vi "Initialization.vi"(8 "error in (no error)":errorcluster, 9 "Init file":string="config_ligne_à_retard.ls", 11 "DelayLineLS4 in":refnum<class "DLLS4.lvclass">) -> (0 "error out":errorcluster, 3 "DelayLineLS4 out":refnum<class "DLLS4.lvclass">)   [LabVIEW 2018, in "DLLS4.lvclass"]
uses:
  DLLS4.lvclass
  C:/Users/Sergey Denisov/Documents/REPS/TRANCON/Classes/GeneralFunctionality/GeneralFunctionality.lvclass
  C:/Users/Sergey Denisov/Documents/REPS/TRANCON/Classes/Delay Line/DelayLine.lvclass
  GeneralFunctionality/GeneralFunctionality.lvclass/GeneralFunctionality.ctl
  DelayLine.lvclass/DelayLine.ctl
  dependecies/globalVarII.vi
  <vilib>/Utility/libraryn.llb/Check if File or Folder Exists.vi
  <vilib>/Utility/error.llb/Error Cluster From Error Code.vi
  Config/Config.lvclass
  DelayLine.lvclass
  GeneralFunctionality/GeneralFunctionality.lvclass
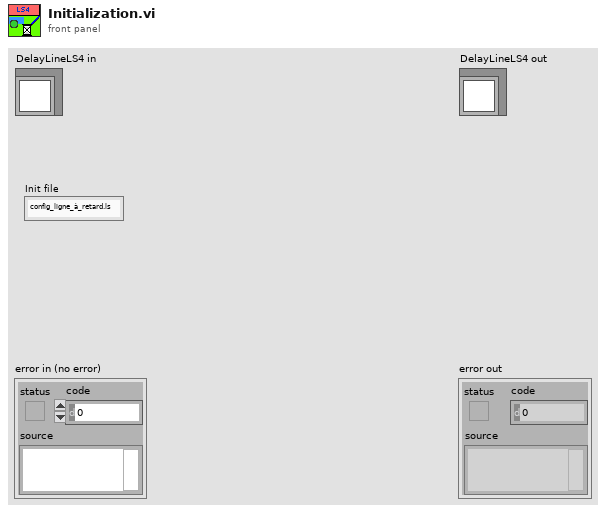
[diagram p1: front panel]
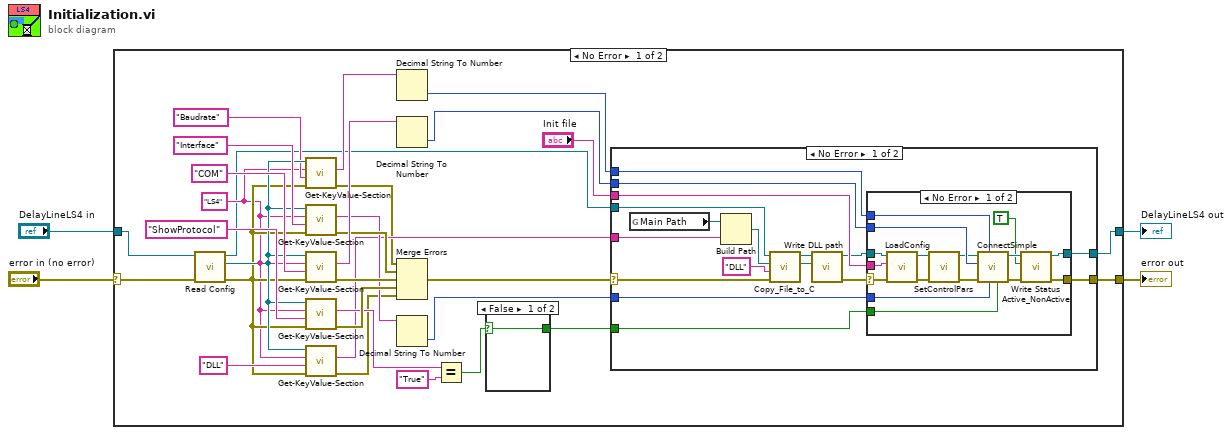
[diagram p0: block diagram]
diagram:
  n1 = case shown="No Error" "error in (no error)" {
    selector: "error in (no error)" -> [w6 w76]
    tunnel: [w35 w76] -> w4
    tunnel: [w34 w75] -> w3
    tunnel: "DelayLineLS4 in" -> [w32 w75]
    frame No Error {
      w9 = "LS4" ("Section")
      n2 = call "Read Config.vi"("error in (no error)"=w6, "GeneralFunctionality en entrée"=w32) -> ("error out"=w12:errorcluster, "Config.lvclass"=w13:refnum<class "Config.lvclass">, "GeneralFunctionality en sortie"=w5:refnum<class "DLLS4.lvclass">)  [unwired: 7 in]
      n3 = call-dynamic "Get-KeyValue-Section.vi"("error in (no error)"=w12, "Key"="Baudrate" ("y"), "Section"=w9, "Config in"=w13) -> ("error out"=w11:errorcluster, "Value"=w8:string)  [unwired: 5 in, 1 out]
      n4 = call-dynamic "Get-KeyValue-Section.vi"("error in (no error)"=w12, "Key"="Interface", "Section"=w9, "Config in"=w13) -> ("error out"=w26:errorcluster, "Value"=w22:string)  [unwired: 5 in, 1 out]
      n5 = call-dynamic "Get-KeyValue-Section.vi"("error in (no error)"=w12, "Key"="COM", "Section"=w9, "Config in"=w13) -> ("error out"=w25:errorcluster, "Value"=w28:string)  [unwired: 5 in, 1 out]
      n6 = call-dynamic "Get-KeyValue-Section.vi"("error in (no error)"=w12, "Key"="ShowProtocol", "Section"=w9, "Config in"=w13) -> ("error out"=w24:errorcluster, "Value"=w20:string)  [unwired: 5 in, 1 out]
      n7 = call-dynamic "Get-KeyValue-Section.vi"("error in (no error)"=w12, "Key"="DLL", "Section"=w9, "Config in"=w13) -> ("error out"=w16:errorcluster, "Value"=w14:string)  [unwired: 5 in, 1 out]
      n8 = Decimal String To Number(string=w8) -> (number=w7:i32)  [unwired: 2 in, 1 out]
      n9 = Decimal String To Number(string=w28) -> (number=w27:i32)  [unwired: 2 in, 1 out]
      n10 = Merge Errors(w11, w26, w25, w24, w16) -> (w23:errorcluster)
      n11 = Decimal String To Number(string=w22) -> (number=w21:i32)  [unwired: 2 in, 1 out]
      n12 = Equal?(x=w20, y="True") -> (x = y?=w18:bool)
      n13 = case shown="False" w18 {
        selector: w18 -> [w36 w37]
        tunnel: [w36 w37] -> w17
        frame False {
        }
        frame True {
        }
      }
      n14 = case shown="No Error" w23 {
        selector: w23 -> [w43 w74]
        tunnel: [w49 w74] -> w35
        tunnel: [w50 w73] -> w34
        tunnel: w5 -> [w42 w73]
        tunnel: "Init file" -> [w54 _]
        tunnel: w21 -> [w53 _]
        tunnel: w27 -> [w52 _]
        tunnel: w17 -> [w51 _]
        tunnel: w14 -> [w45 _]
        tunnel: w7 -> [w44 _]
        frame No Error {
          n15 = global read "globalVarII.vi" "Main Path"() -> (w48:path)
          n16 = Build Path(base path=w48, name or relative path=w45) -> (appended path=w39:path)
          n17 = call "Copy_File_to_C.vi"("error in (no error)"=w43, "Folder"="DLL", "path from"=w39, "GeneralFunctionality in"=w42) -> ("appended path out"=w40:path, "GeneralFunctionality out"=w41:refnum<class "DLLS4.lvclass">)  [unwired: 5 in, 1 out]
          n18 = call "Write DLL path.vi"("DLL path"=w40, "DelayLine in"=w41) -> ("error out"=w46:errorcluster, "DelayLine out"=w47:refnum<class "DLLS4.lvclass">)  [unwired: 8 in]
          n19 = case shown="No Error" w46 {
            selector: w46 -> [w55 w71]
            tunnel: w54 -> [w65 _]
            tunnel: w53 -> [w70 _]
            tunnel: w52 -> [w69 _]
            tunnel: w51 -> [w68 _]
            tunnel: [w67 w72] -> w50
            tunnel: [w66 w71] -> w49
            tunnel: w47 -> [w56 w72]
            tunnel: w44 -> [w64 _]
            frame No Error {
              n20 = call "LoadConfig.vi"("error in (no error)"=w55, "FileName"=w65, "DelayLineLS4 in"=w56) -> ("error out"=w60:errorcluster, "DelayLineLS4 out"=w63:refnum<class "DLLS4.lvclass">)  [unwired: 7 in]
              n21 = call "SetControlPars.vi"("error in (no error)"=w60, "DelayLineLS4 in"=w63) -> ("error out"=w59:errorcluster, "DelayLineLS4 out"=w62:refnum<class "DLLS4.lvclass">)  [unwired: 8 in]
              n22 = call "ConnectSimple.vi"("Show Protocol"=w68, "Interface (1: RS232; 2: ArcNet; 3: DPRAM)"=w70, "Baudrate"=w64, "error in (no error)"=w59, "COM Port"=w69, "DelayLineLS4 in"=w62) -> ("error out"=w58:errorcluster, "DelayLineLS4 out"=w61:refnum<class "DLLS4.lvclass">)  [unwired: 4 in]
              n23 = call "Write Status Active_NonActive.vi"("error in (no error)"=w58, "Status Active/NonActive"=TRUE, "GeneralFunctionality in"=w61) -> ("error out"=w66:errorcluster, "GeneralFunctionality out"=w67:refnum<class "DLLS4.lvclass">)  [unwired: 7 in]
            }
            frame Error {
            }
          }
        }
        frame Error {
        }
      }
    }
    frame Error {
    }
  }
  "error out" <- w4
  "DelayLineLS4 out" <- w3
